vi "train.vi"(1 "error in (no error)":errorcluster, 2 "weight_normalization":bool, 3 "Conjugate":bool, 4 "ptr":i64, 5 "batch_update":u32, 6 "input":sgl[][](array[numeric]), 7 "eta":sgl, 9 "outputDesired":sgl[][](array[numeric]), 11 "adam":bool, 12 "lambda":sgl) -> (13 "prediction":sgl[][](array[numeric]), 15 "error out":errorcluster, 18 "ptr out":i64, 19 "error":sgl)   [LabVIEW 2016, in "CNet.lvlib"]
uses:
  CNet.lvlib
  Users/jg754/Documents/Visual Studio 2015/Projects/CLearn/x64/Debug/CLearn.dll
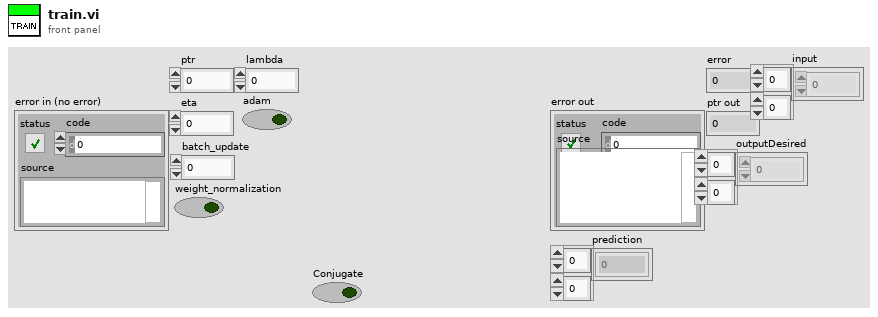
[diagram p1: front panel]
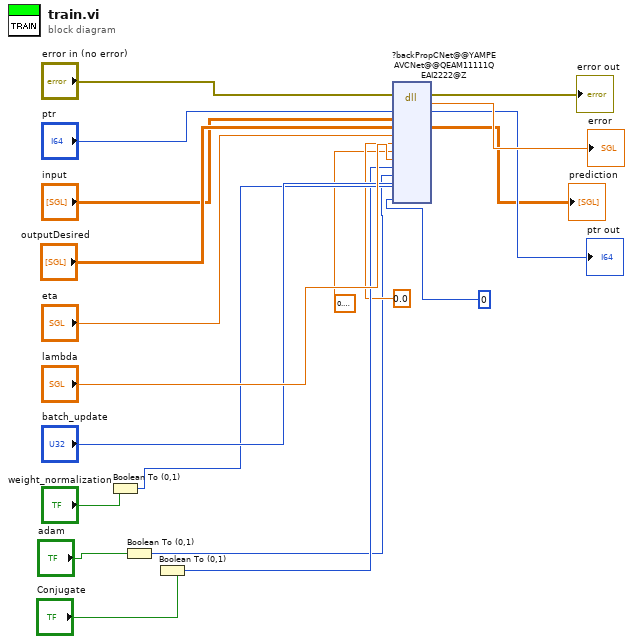
[diagram p0: block diagram]
diagram:
  n1 = Boolean To (0,1)(Boolean="weight_normalization") -> (0, 1=w11:i16)
  n2 = Boolean To (0,1)(Boolean="adam") -> (0, 1=w1:i16)
  n3 = Boolean To (0,1)(Boolean="Conjugate") -> (0, 1=w10:i16)
  n4 = dll-call lib="C:/Users/jg754/Documents/Visual Studio 2015/Projects/CLearn/x64/Debug/CLearn.dll" fn="?backPropCNet@@YAMPEAVCNet@@QEAM11111QEAI2222@Z"(error in="error in (no error)", "ptr"="ptr", "input"="input", "outputDesired"="outputDesired", "eta"="eta", "metaEta"=sgl 0.0, "gamma"=sgl 0.9, "lambda"="lambda", "conjugate"=w10, "adam"=w1, "batch_update"="batch_update", "weight_normalization"=w11, "initializationPass"=u32 0) -> (error out=→"error out":errorcluster, "error"=→"error":sgl, "ptr"=→"ptr out":i64, "outputDesired"=→"prediction":sgl[][])  [unwired: 12 in, 1 out]
